vi "Encoder scales.vi"() -> ()   [LabVIEW 2017]
panel:
  out "Numeric Control 2":i16
  out "x/y":i16
  in  "40":i16
  in  "Numeric Control":i16
  out "High throughput sin & cos scale":ext=5.555555555555556e-05
  in  "encoding method 2":ext=4.0
  in  "gearhead ratio 2":ext=35.0
  in  "small bevel gear  2":ext=24.0
  in  "pulses per rev. 2":ext=1024.0
  out "ENC_2_SCALE":ext=0.2197265625
  in  "big bevel gear 2":ext=48.0
  in  "big spur gear":ext=80.0
  out "ENC_1_SCALE":ext=0.2197265625
  in  "pulses per rev.":ext=1024.0
  in  "small spur gear":ext=30.0
  in  "gearhead ratio":ext=15.0
  in  "encoding method":ext=4.0
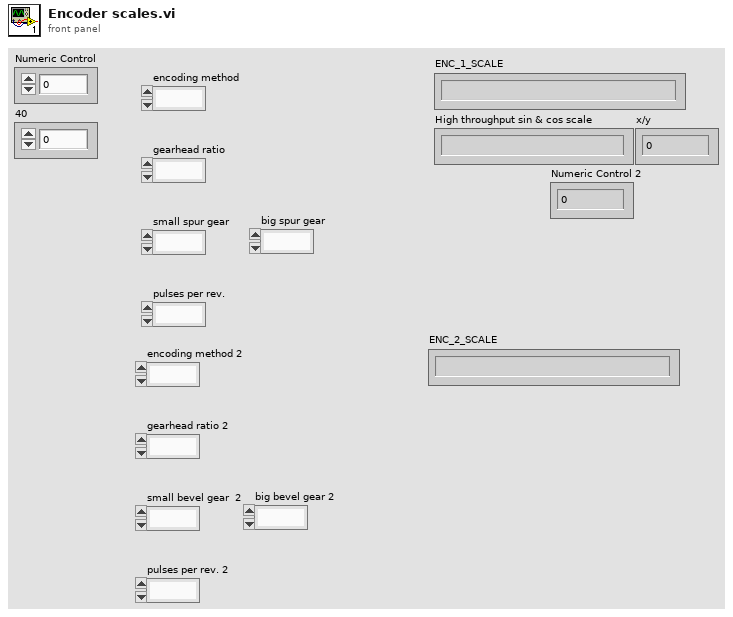
[diagram p1: front panel]
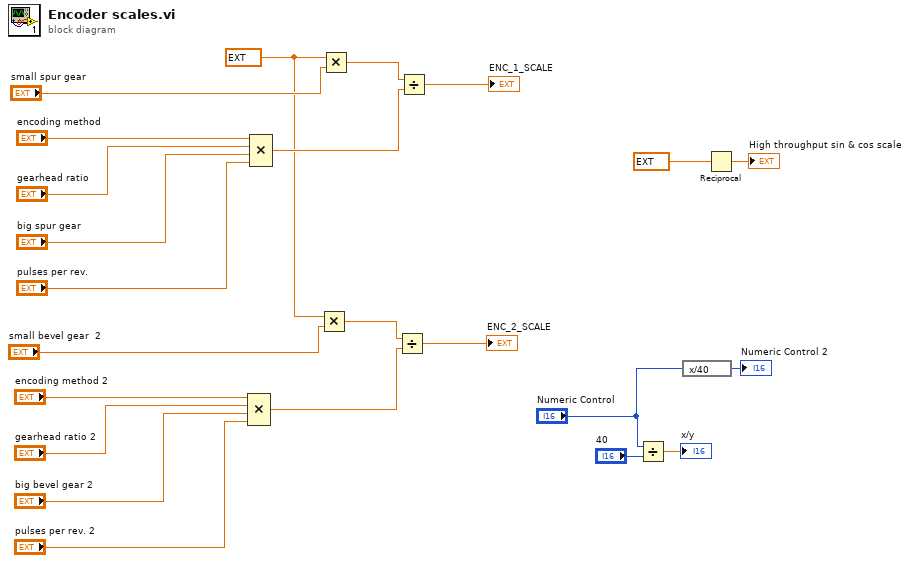
[diagram p0: block diagram]
diagram:
  w1 = ext 36000.0
  n1 = Compound Arithmetic op=MULTIPLY("encoding method 2", "gearhead ratio 2", "big bevel gear 2", "pulses per rev. 2") -> (w15:ext)
  n2 = Compound Arithmetic op=MULTIPLY("encoding method", "gearhead ratio", "big spur gear", "pulses per rev.") -> (w16:ext)
  n3 = Multiply(x=w1, y="small bevel gear  2") -> (x*y=w14:ext)
  n4 = Multiply(x=w1, y="small spur gear") -> (x*y=w17:ext)
  n5 = Divide(x=w14, y=w15) -> (x/y=→"ENC_2_SCALE":ext)
  n6 = Divide(x=w17, y=w16) -> (x/y=→"ENC_1_SCALE":ext)
  n7 = Divide(x="Numeric Control", y="40") -> (x/y=→"x/y":dbl)
  n8 = expression code="x/40"("Numeric Control") -> (→"Numeric Control 2":i16)
  n9 = Reciprocal(x=ext 18000.0) -> (1/x=→"High throughput sin & cos scale":ext)
